vi "Background Loop.vi"(8 "error in (no error)":errorcluster, 10 "Action":T1, 11 "Worker in":refnum<class "Worker.lvclass">) -> (0 "error out":errorcluster, 3 "Worker out":refnum<class "Worker.lvclass">, 4 "Result":refnum<class "Acquired Result.lvclass">)   [LabVIEW 2021, in "Worker.lvclass"]
uses:
  Worker.lvclass
  Worker.lvclass/Worker.ctl
  Worker Messages/Background Loop Msg/Background Loop Msg.lvclass
  <vilib>/ActorFramework/Actor/Actor.lvclass
  C:/Program Files/National Instruments/LabVIEW 2021/vi.lib/ActorFramework/Actor/Actor.lvclass
  C:/Program Files/National Instruments/LabVIEW 2021/vi.lib/ActorFramework/Message/Message.lvclass
  Background Loop Action.ctl
  NHMFL_Core/Libraries/Instruments/Results/Acquired Result/Acquired Result.lvclass
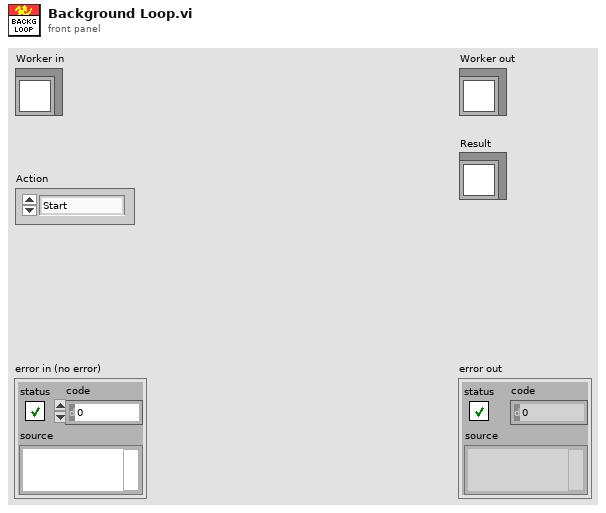
[diagram p1: front panel]
types:
  T1 = typedef "Background Loop Action.ctl" = enum16{"Start", "Continue", "Stop"}
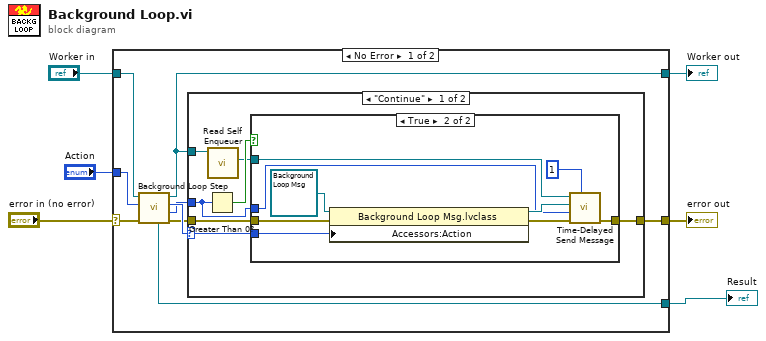
[diagram p0: block diagram]
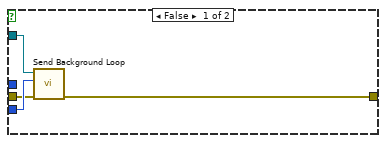
[diagram p2: hidden frame]
diagram:
  n1 = case shown="No Error" "error in (no error)" {
    selector: "error in (no error)" -> [w14 w38]
    tunnel: [w9 w38] -> w5
    tunnel: [w11 w37] -> w3
    tunnel: "Worker in" -> [w15 w37]
    tunnel: "Action" -> [w8 _]
    tunnel: [w7 _] -> w1
    frame No Error {
      n2 = call-dynamic "Background Loop Step.vi"("error in (no error)"=w14, "Action"=w8, "Worker in"=w15) -> ("error out"=w10:errorcluster, "Next step delay"=w12:i32, "Action out"=w13:T1, "Worker out"=w11:refnum<class "Worker.lvclass">, "Result"=w7:refnum<class "Acquired Result.lvclass">)  [unwired: 4 in]
      n3 = case shown="\"Continue\"" w13 {
        selector: w13 -> [w22 _]
        tunnel: w12 -> [w16 _]
        tunnel: w11 -> [w20 _]
        tunnel: w10 -> [w19 w36]
        tunnel: [w17 w36] -> w9
        frame "Continue" {
          n4 = Greater Than 0?(x=w16) -> (x > 0?=w21:bool)
          n5 = call <vilib>:"Read Self Enqueuer.vi"("Actor"=w20) -> ("Self Enqueuer"=w18:refnum<class "Message Enqueuer.lvclass">)  [unwired: 10 in]
          n6 = case shown="True" w21 {
            tunnel: w22 -> [w25 w34]
            tunnel: w19 -> [w24 w32]
            tunnel: w18 -> [w26 w28]
            tunnel: [w23 w29] -> w17
            tunnel: w16 -> [_ w31]
            frame False {
              n7 = call "Send Background Loop.vi"("error in (no error)"=w24, "Action"=w25, "Message Enqueuer"=w26) -> ("error out"=w23:errorcluster)  [unwired: 7 in, 1 out]
            }
            frame True {
              n8 = property class="Background Loop Msg.lvclass"(reference=refnum<class "Background Loop Msg.lvclass"> refnum ("Background Loop Msg.lvclass"), error in=w32, "Accessors:Action"=w34) -> (reference out=w33:refnum<class "Background Loop Msg.lvclass">, error out=w30:errorcluster)
              n9 = call <vilib>:"Time-Delayed Send Message.vi"("# Copies (0 = infinite repeat)"=u32 1, "error in (no error)"=w30, "Milliseconds To Wait"=w31, "Message"=w33, "Message Enqueuer"=w28) -> ("error out"=w29:errorcluster)  [unwired: 5 in, 1 out]
            }
          }
        }
        frame "Stop", Default {
        }
      }
    }
    frame Error {
    }
  }
  "error out" <- w5
  "Worker out" <- w3
  "Result" <- w1
